vi "Delta JSON Update.vi"(10 "Delta JSON":string, 11 "JSON string in":string) -> (3 "JSON string out":string)   [LabVIEW 2019]
uses:
  <vilib>/MultiError/TokenizeJSON/Multi Error Cluster.lvlib
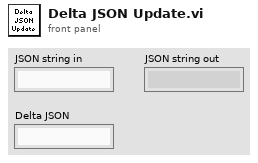
[diagram p1: front panel]
types:
  T1 = cluster{"whole match":string, "orig":i32, "delta":i32}[]
  T2 = typedef "Multi Error Cluster.lvlib/JSON Token Descriptor.ctl" = cluster{"match string":string, "raw token type":T3, "byte offset ":i32}
  T3 = typedef "Multi Error Cluster.lvlib/JSON Raw Token Values.ctl" = enum32{"{", "}", "[", "]", ",", ":", "\"", "number", "string", "true", "false", "null", "invalid"}
  T4 = typedef "Multi Error Cluster.lvlib/JSON Token Values.ctl" = enum32{"array begin", "array end", "object begin", "object end", "value", "invalid", "name"}
  T5 = cluster{"whole match":string, "token index":i32}[]
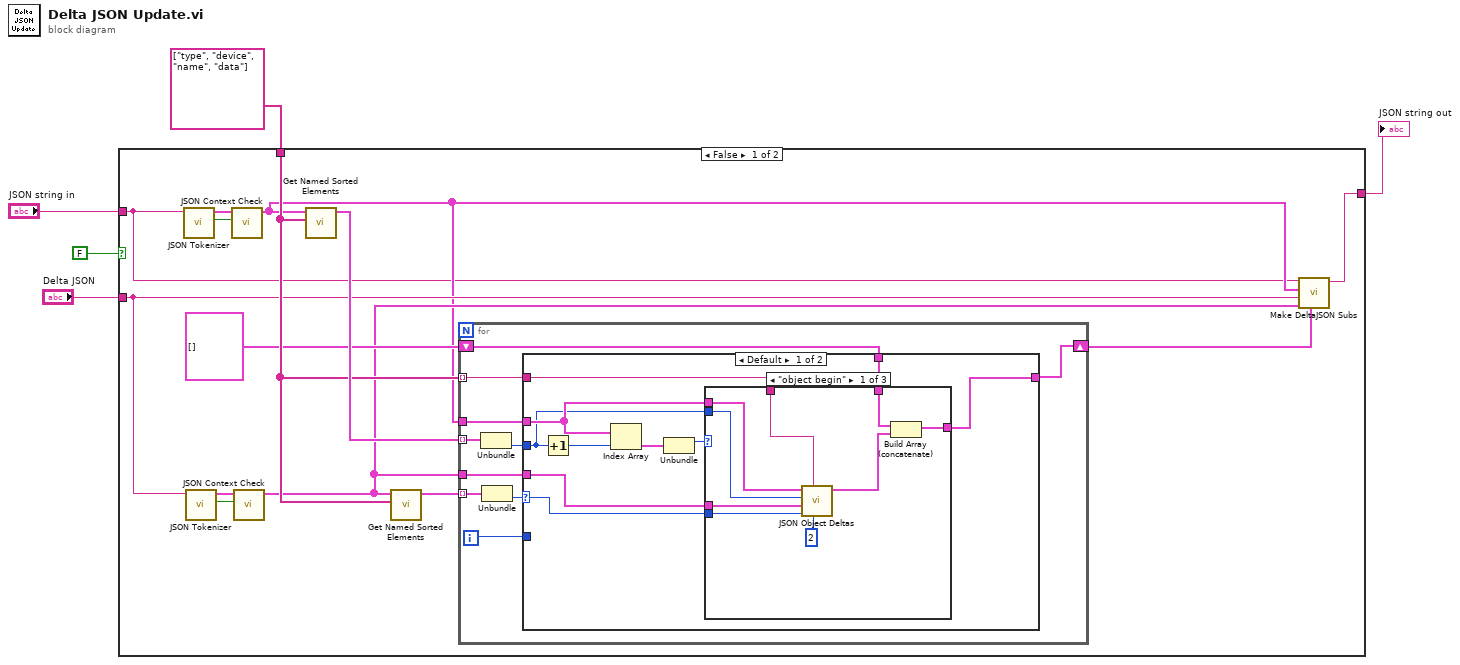
[diagram p0: block diagram]
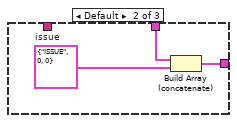
[diagram p2: hidden frame]
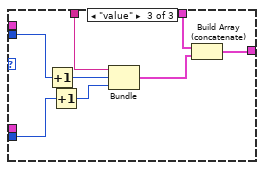
[diagram p3: hidden frame]
diagram:
  n1 = case shown="False" FALSE {
    tunnel: "JSON string in" -> [w6 w61]
    tunnel: [w7 w61] -> w2
    tunnel: "Delta JSON" -> [w11 _]
    tunnel: string[] ["type", "device", "name", "data"] ("names") -> [w13 _]
    frame False {
      n2 = call <vilib>:"JSON Tokenizer.vi"("JSON String"=w6) -> ("Invalid"=w18:bool, "Array"=w19:T2[])  [unwired: 9 in]
      n3 = call <vilib>:"JSON Tokenizer.vi"("JSON String"=w11) -> ("Invalid"=w17:bool, "Array"=w16:T2[])  [unwired: 9 in]
      n4 = call <vilib>:"JSON Context Check.vi"("Invalid in"=w18, "Parse Tokens in"=w19) -> ("tokens"=w8:cluster{"token type":T4, T2}[])  [unwired: 8 in, 1 out]
      n5 = call <vilib>:"JSON Context Check.vi"("Invalid in"=w17, "Parse Tokens in"=w16) -> ("tokens"=w9:cluster{"token type":T4, T2}[])  [unwired: 8 in, 1 out]
      n6 = call "Get Named Sorted Elements.vi"("names"=w13, "tokens"=w8) -> ("sorted info"=w14:T5)  [unwired: 9 in]
      n7 = call "Get Named Sorted Elements.vi"("names"=w13, "tokens"=w9) -> ("sorted info"=w15:T5)  [unwired: 9 in]
      n8 = for {
        tunnel: w15 -> [w29] mode=indexing
        tunnel: w14 -> [w27] mode=indexing
        tunnel: w8 -> [w26]
        tunnel: w9 -> [w25]
        shift-right: [w23] -> w10
        shift-left: T1 [] -> [w22]
        tunnel: w13 -> [w21] mode=indexing
        i -> [w20]
        n9 = Unbundle(w27) -> ("token index"=w24:i32)  [unwired: 1 out]
        n10 = Unbundle(w29) -> ("token index"=w28:i32)  [unwired: 1 out]
        n11 = case shown="Default" w28 {
          selector: w28 -> [w31 _]
          tunnel: w26 -> [w33 _]
          tunnel: w25 -> [w32 _]
          tunnel: w24 -> [w30 _]
          tunnel: [w34 w60] -> w23
          tunnel: w22 -> [w35 w60]
          tunnel: w21 -> [w39 _]
          tunnel: w20 -> [_ _]
          frame Default {
            n12 = Increment(x=w30) -> (x+1=w38:i32)
            n13 = Index Array(array=w33, index=w38) -> (element=w37:cluster{"token type":T4, T2})
            n14 = Unbundle(w37) -> ("token type"=w36:T4)  [unwired: 1 out]
            n15 = case shown="\"object begin\"" w36 {
              tunnel: w39 -> [w48 _ w59]
              tunnel: w35 -> [w47 w51 w58]
              tunnel: [w45 w49 w56] -> w34
              tunnel: w33 -> [w41 _ _]
              tunnel: w32 -> [w43 _ _]
              tunnel: w31 -> [w44 _ w52]
              tunnel: w30 -> [w42 _ w53]
              frame "object begin" {
                n16 = call "JSON Object Deltas.vi"("index  offset"=2, "name"=w48, "delta index"=w44, "delta tokens"=w43, "full index"=w42, "full tokens"=w41) -> ("Subs"=w46:T1)  [unwired: 5 in]
                n17 = Build Array (concatenate)(w47, w46) -> (w45:T1)
              }
              frame Default {
                w50 = cluster{"whole match":string, i32, i32} {"whole match"="ISSUE", 0, 0}  # issue
                n18 = Build Array (concatenate)(w51, w50) -> (w49:T1)
              }
              frame "value" {
                n19 = Increment(x=w53) -> (x+1=w54:i32)
                n20 = Increment(x=w52) -> (x+1=w55:i32)
                n21 = Bundle("whole match"=w59, w54, w55) -> (w57:cluster{"whole match":string, i32, i32})  [unwired: 1 in]
                n22 = Build Array (concatenate)(w58, w57) -> (w56:T1)
              }
            }
          }
          frame -1 {
          }
        }
      }
      n23 = call "Make DeltaJSON Subs.vi"("Array"=w10, "delta"=w9, "Delta JSON"=w11, "orig"=w8, "orig string"=w6) -> ("result string"=w7:string)  [unwired: 6 in]
    }
    frame True {
    }
  }
  "JSON string out" <- w2
